vi "dfd_Parse Subband Filters from XML String.vi"(8 "error in":errorcluster, 10 "string in":string, 11 "filter banks":T1={"mFBank_AnalysisFilters"=[], "mFBank_SynthesisFilters"=[], "mFBank_#Bands"=2, "mFBank_ProcMethod"=enum."General", "mFBank_Coeffs"=[], "mFBank_Gain"=1.0, "mFBank_Delay"=0, "mFBank_Type"=0} {"mFBank_SynthesisFilters"."mMRate_SumWl" min=1 max=32 step=1; "mFBank_SynthesisFilters"."mMRate_InputIwl" min=1 max=32 step=1; "mFBank_SynthesisFilters"."mMRate_GainWl" min=1 max=32 step=1; "mFBank_SynthesisFilters"."mMRate_OutputWl" min=1 max=32 step=1; "mFBank_SynthesisFilters"."mMRate_InputWl" min=1 max=32 step=1; "mFBank_SynthesisFilters"."mMRate_CoefWl" min=1 max=32 step=1; "mFBank_SynthesisFilters"."mMRate_Mode" items=["Default"=-1, "No Rate Change"=0, "Interpolation"=1, "Decimation"=2, "Interpolated"=3, "Rational"=4]; "mFBank_AnalysisFilters"."mMRate_SumWl" min=1 max=32 step=1; "mFBank_AnalysisFilters"."mMRate_InputIwl" min=1 max=32 step=1; "mFBank_AnalysisFilters"."mMRate_GainWl" min=1 max=32 step=1; "mFBank_AnalysisFilters"."mMRate_OutputWl" min=1 max=32 step=1; "mFBank_AnalysisFilters"."mMRate_InputWl" min=1 max=32 step=1; "mFBank_AnalysisFilters"."mMRate_CoefWl" min=1 max=32 step=1; "mFBank_AnalysisFilters"."mMRate_Mode" items=["Default"=-1, "No Rate Change"=0, "Interpolation"=1, "Decimation"=2, "Interpolated"=3, "Rational"=4]; "mFBank_Type" items=["Uniform", "Non-Uniform"]}) -> (0 "error out":errorcluster, 2 "dup string":string, 3 "filter banks out":T1={"mFBank_AnalysisFilters"=[], "mFBank_SynthesisFilters"=[], "mFBank_#Bands"=2, "mFBank_ProcMethod"=enum."General", "mFBank_Coeffs"=[], "mFBank_Gain"=1.0, "mFBank_Delay"=0, "mFBank_Type"=0} {"mFBank_SynthesisFilters"."mMRate_SumWl" min=1 max=32 step=1; "mFBank_SynthesisFilters"."mMRate_InputIwl" min=1 max=32 step=1; "mFBank_SynthesisFilters"."mMRate_GainWl" min=1 max=32 step=1; "mFBank_SynthesisFilters"."mMRate_OutputWl" min=1 max=32 step=1; "mFBank_SynthesisFilters"."mMRate_InputWl" min=1 max=32 step=1; "mFBank_SynthesisFilters"."mMRate_CoefWl" min=1 max=32 step=1; "mFBank_SynthesisFilters"."mMRate_Mode" items=["Default"=-1, "No Rate Change"=0, "Interpolation"=1, "Decimation"=2, "Interpolated"=3, "Rational"=4]; "mFBank_AnalysisFilters"."mMRate_SumWl" min=1 max=32 step=1; "mFBank_AnalysisFilters"."mMRate_InputIwl" min=1 max=32 step=1; "mFBank_AnalysisFilters"."mMRate_GainWl" min=1 max=32 step=1; "mFBank_AnalysisFilters"."mMRate_OutputWl" min=1 max=32 step=1; "mFBank_AnalysisFilters"."mMRate_InputWl" min=1 max=32 step=1; "mFBank_AnalysisFilters"."mMRate_CoefWl" min=1 max=32 step=1; "mFBank_AnalysisFilters"."mMRate_Mode" items=["Default"=-1, "No Rate Change"=0, "Interpolation"=1, "Decimation"=2, "Interpolated"=3, "Rational"=4]; "mFBank_Type" items=["Uniform", "Non-Uniform"]})   [LabVIEW 2017, in "NI_DigFilter_FilterBank.lvlib"]
uses:
  <vilib>/addons/Digital Filter Design/NI_DigFilter_FilterBank.lvlib
  <vilib>/addons/Digital Filter Design/FilterBank.llb/Object/DFD Filter Bank Obj.ctl
  <vilib>/addons/Digital Filter Design/_Objects.llb/DFD Multirate Filter Obj.ctl
  <vilib>/addons/Digital Filter Design/_Objects.llb/DFD Multirate Mode.ctl
  <vilib>/addons/Digital Filter Design/_Objects.llb/DFD Coef Norm Type.ctl
  <vilib>/addons/Digital Filter Design/_Objects.llb/DFD Round-off Mode.ctl
  <vilib>/addons/Digital Filter Design/_Objects.llb/DFD FXP MRate Multiply Mode.ctl
  <vilib>/addons/Digital Filter Design/FilterBank.llb/Object/DFD Filter Bank Processing Method.ctl
  <vilib>/addons/Digital Filter Design/FilterBank.llb/Object/DFD Filter Bank Type.ctl
  <vilib>/addons/Digital Filter Design/NI_DigFilterLicensed.lvlib
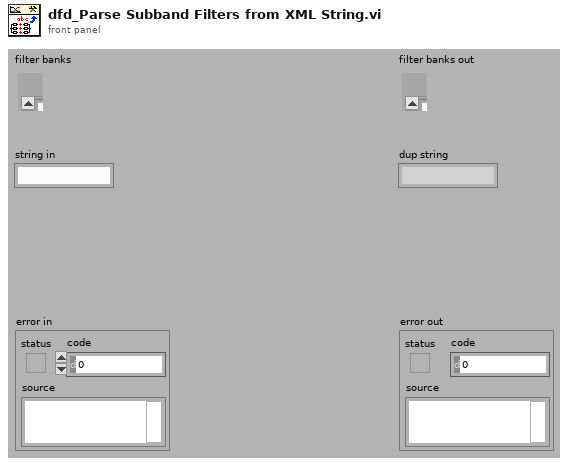
[diagram p1: front panel]
types:
  T1 = typedef "NI_DigFilter_FilterBank.lvlib/DFD Filter Bank Obj.ctl" = cluster{"mFBank_AnalysisFilters":T2[], "mFBank_SynthesisFilters":T2[], "mFBank_#Bands":i32, "mFBank_ProcMethod":T7, "mFBank_Coeffs":dbl[], "mFBank_Gain":dbl, "mFBank_Delay":i32, "mFBank_Type":T8}
  T2 = typedef "NI_DigFilterLicensed.lvlib/DFD Multirate Filter Obj.ctl" = cluster{"mMRate_Structure":enum16{"CIC", "FIR", "IIR", "Lattice"}, "mMRate_Mode":T3, "mMRate_Factor":i32, "mMRate_FIRParams":cluster{"mMRate_FIR_H":dbl[], "mMRate_FIR_IsNyquist?":bool, "mMRate_FIR_IsSymmetric?":bool}, "mMRate_CICParams":cluster{"mMRate_CIC_#Stage":i32, "mMRate_CIC_Lag":i32, "mMRate_CIC_Type":enum16{"Lowpass", "Highpass"}}, "mMRate_Order":i32, "mMRate_Version":string, "mMRate_Comments":string, "mMRate_RationalFactor":cluster{"mMRate_L":i32, "mMRate_M":i32}, "mMRate_Fs":dbl, "mMRate_Quantized?":bool, "mMRate_QFilterGain":dbl, "mMRate_CoefWl":i16, "mMRate_Scaling":cluster{"mMRate_ScaleByPowerOf2?":bool, "mMRate_ScaleType":T4}, "mMRate_InputWl":i16, "mMRate_OutputWl":i16, "mMRate_OutputMode":T5, "mMRate_MultMode":T6, "mMRate_BitPruning":bool, "mMRate_GainWl":i16, "mMRate_OutputFwl":i16, "mMRate_SumIwl":i16, "mMRate_InputIwl ":i16, "mMRate_SumWl":i16, "mMRate_CoefIwl":i16}
  T3 = typedef "NI_DigFilterLicensed.lvlib/DFD Multirate Mode.ctl" = i16
  T4 = typedef "NI_DigFilterLicensed.lvlib/DFD Coef Norm Type.ctl" = enum16{"No Norm", "Time Domain 1-Norm", "Time Domain 2-Norm", "Time Domain Inf-Norm"}
  T5 = typedef "NI_DigFilterLicensed.lvlib/DFD Round-off Mode.ctl" = enum16{"Nearest", "Truncation"}
  T6 = typedef "NI_DigFilterLicensed.lvlib/DFD FXP MRate Multiply Mode.ctl" = enum16{"Truncated", "Full"}
  T7 = typedef "NI_DigFilter_FilterBank.lvlib/DFD Filter Bank Processing Method.ctl" = enum16{"General", "2-Band QMF Lattice", "Cosine-Modulated"}
  T8 = typedef "NI_DigFilter_FilterBank.lvlib/DFD Filter Bank Type.ctl" = u16
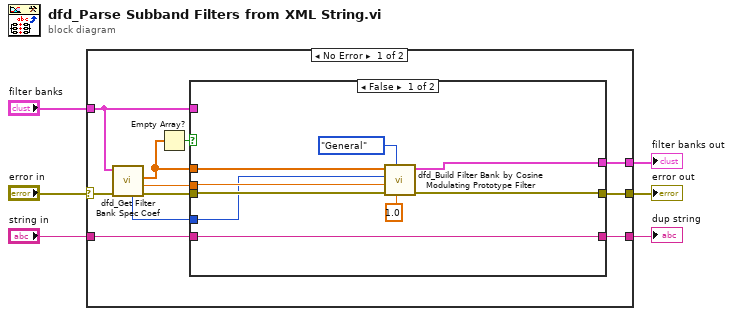
[diagram p0: block diagram]
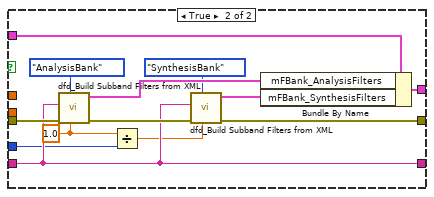
[diagram p2: hidden frame]
diagram:
  n1 = case shown="No Error" "error in" {
    selector: "error in" -> [w13 w41]
    tunnel: "string in" -> [w15 w40]
    tunnel: [w16 w41] -> w4
    tunnel: [w17 _] -> w3
    tunnel: "filter banks" -> [w14 _]
    tunnel: [w9 w40] -> w1
    frame No Error {
      n2 = call <vilib>:"dfd_Get Filter Bank Spec Coef.vi"("error in (no error)"=w13, "filter bank"=w14) -> ("error out"=w12:errorcluster, "gain"=w8:dbl, "coefficients"=w10:dbl[], "number of bands"=w7:i32)  [unwired: 4 in, 2 out]
      n3 = Empty Array?(array=w10) -> (empty?=w11:bool)
      n4 = case shown="False" w11 {
        tunnel: [w23 w38] -> w17
        tunnel: [w22 w33] -> w16
        tunnel: w15 -> [w21 w30]
        tunnel: w14 -> [_ w32]
        tunnel: w12 -> [w19 w31]
        tunnel: w10 -> [w26 _]
        tunnel: [w21 w30] -> w9
        tunnel: w8 -> [w20 _]
        tunnel: w7 -> [w18 w28]
        frame False {
          n5 = call <vilib>:"dfd_Build Filter Bank by Cosine Modulating Prototype Filter.vi"("fs in [Hz]"=1.0, "processing method"=DFD_Filter_Bank_Processing_Method."General", "error in"=w19, "gain"=w20, "band counts"=w18, "filter coefficients"=w26) -> ("error out"=w22:errorcluster, "filter bank out"=w23:T1)  [unwired: 4 in]
        }
        frame True {
          w29 = 1.0 ("fs")
          n6 = call <vilib>:"dfd_Build Subband Filters from XML.vi"("fs"=w29, "Bank"=enum16{"AnalysisBank", "SynthesisBank"}."AnalysisBank", "error in"=w31, "content"=w30) -> ("error out"=w36:errorcluster, "subband filters"=w39:T2[])  [unwired: 5 in, 1 out]
          n7 = Divide(x=w29, y=w28) -> (x/y=w27:dbl)
          n8 = call <vilib>:"dfd_Build Subband Filters from XML.vi"("fs"=w27, "Bank"=enum16{"AnalysisBank", "SynthesisBank"}."SynthesisBank", "error in"=w36, "content"=w30) -> ("error out"=w33:errorcluster, "subband filters"=w34:T2[])  [unwired: 5 in, 1 out]
          n9 = Bundle By Name(cluster=w32, "mFBank_AnalysisFilters"=w39, "mFBank_SynthesisFilters"=w34) -> (w38:T1)
        }
      }
    }
    frame Error {
    }
  }
  "dup string" <- w1
  "error out" <- w4
  "filter banks out" <- w3
